vi "Battery_Destroy.vi"(0 "reference in":refnum<class "Battery.lvclass">, 5 "Error In":errorcluster) -> (14 "reference out":refnum<class "Battery.lvclass">, 19 "Error Out":errorcluster)   [LabVIEW 2023, in "Battery.lvclass"]
uses:
  Battery.lvclass
  Battery.lvclass/Battery.ctl
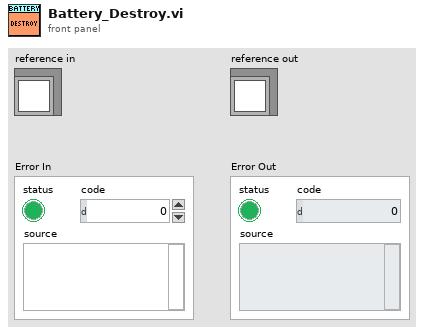
[diagram p1: front panel]
types:
  T1 = typedef "Battery.lvclass/ObjectAttributes.ctl" = cluster{"Python module":path, "Python Session":refnum<k35>, "PybammWrapper":refnum<k38>, "model loaded":bool, "simulation loaded":bool, "simulation enabled":bool, "SOC OCV Curve":dbl[][], "Open Circuit Voltage (V)":dbl, "State of Charge (%)":dbl, "# Cells in Series":u16, "# Cells in Parallel":u16, "Model Parameters":T2, "Simulation Parameters":T3, "Power Module":refnum<class "PowerModuleInterface.lvclass">}
  T2 = typedef "Battery.lvclass/Model Parameters.ctl" = cluster{"chemistry":string, "model_type":string}
  T3 = typedef "Battery.lvclass/Simulation Parameters.ctl" = cluster{"num_rc_pairs":i32, "R0":dbl, "R1":dbl, "C1":dbl, "R2":dbl, "C2":dbl, " nominal_capacity_Ah":dbl, "upper_voltage_cutoff":dbl, "lower_voltage_cutoff":dbl}
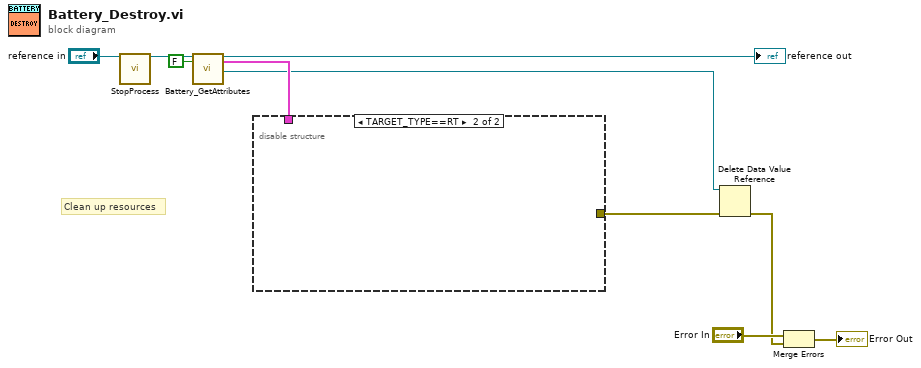
[diagram p0: block diagram]
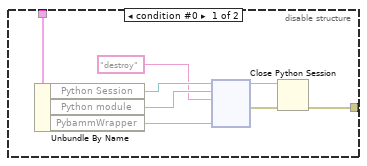
[diagram p2: hidden frame]
diagram:
  # "Clean up resources"
  n1 = call "StopProcess.vi"("reference in"="reference in") -> ("reference out"=w7:refnum<class "Battery.lvclass">)  [unwired: 17 in, 1 out]
  n2 = call "Battery_GetAttributes.vi"("reference in"=w7, "OnlyGetDvrReference(False)"=FALSE) -> ("reference out"=→"reference out":refnum<class "Battery.lvclass">, "Data"=w4:T1, "DataRef"=w2:refnum<data-value>)  [unwired: 14 in, 1 out]
  n3 = disable-structure shown="TARGET_TYPE==RT" {
    disable-tunnel: w4 -> [w18 _]
    disable-tunnel: [w15 _] -> w3
    frame condition #0 {
      n4 = Unbundle By Name(w18) -> ("Python Session"=w17:refnum<k35>, "Python module"=w16:path, "PybammWrapper"=w14:refnum<k38>)
      n5 = node(w17, w16, "destroy" ("function name"), w14) -> (w11:refnum<k35>, w12:errorcluster)  [unwired: 4 in, 2 out]
      n6 = Close Python Session(session in=w11, error in=w12) -> (11:w15:errorcluster)
    }
    frame condition #1 (active) {
    }
  }
  n7 = Delete Data Value Reference(data value reference=w2, error in=w3) -> (error out=w1:errorcluster)  [unwired: 1 out]
  n8 = Merge Errors("Error In", w1) -> (→"Error Out":errorcluster)
